vi "Configure Multi Eval Meas Modulation IQ Enabled.vi"(8 "error in (no error)":errorcluster, 9 "IQ Enabled (On)":bool=TRUE, 10 "Instance (1)":i32=1, 11 "VISA resource name":refnum<visa-resource-name>) -> (0 "error out":errorcluster, 3 "VISA resource name out":refnum<visa-resource-name>)   [LabVIEW 2015, in "Rohde&Schwarz CMP LR WPAN Measurement.lvlib"]
doc: "Enables or disables the evaluation of IQ results in the multi-evaluation measurement.\n\nAttribute:\nRSCMPLRWM_ATTR_MULTIEVAL_MODULATION_IQ_ENABLED\n\nRemote-control command:\nCONFigure:WPAN:MEAS<i>:MEValuation:RESult:IQ"
uses:
  <instrlib>/Rohde&Schwarz CMP LR WPAN Measurement/Rohde&Schwarz CMP LR WPAN Measurement.lvlib
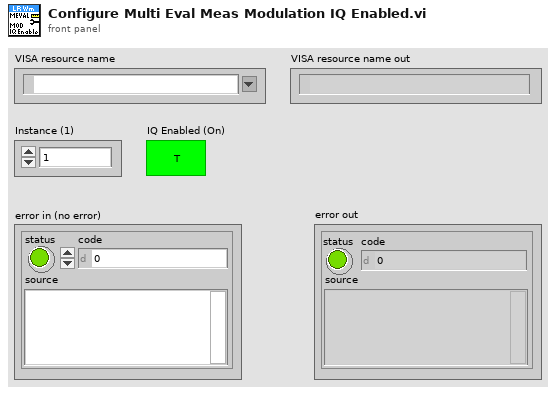
[diagram p1: front panel]
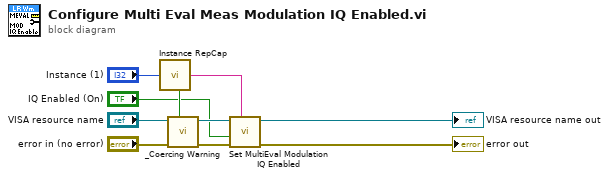
[diagram p0: block diagram]
diagram:
  n1 = call <instrlib>:"Instance RepCap.vi"("Instance In"="Instance (1)") -> ("In Range?"=w8:bool, "RepCap Identifier Out"=w7:string)  [unwired: 1 in]
  n2 = call <instrlib>:"_Coercing Warning.vi"("In Range?"=w8, "error in (no error)"="error in (no error)", "VISA resource name"="VISA resource name") -> ("error out"=w4:errorcluster, "VISA resource name out"=w3:refnum<visa-resource-name>)  [unwired: 7 in]
  n3 = call "Set MultiEval Modulation IQ Enabled"("Repeated Capabilities"=w7, "error in (no error)"=w4, "MultiEval Modulation IQ Enabled (OFF)"="IQ Enabled (On)", "instrument handle"=w3) -> ("error out"=→"error out":errorcluster, "instrument handle out"=→"VISA resource name out":refnum<visa-resource-name>)  [unwired: 6 in]
